vi "verify.vi"(8 "error in":errorcluster, 11 "connection ID":i32) -> (0 "error out":errorcluster, 3 "connection ID":i32)   [LabVIEW 2016]
doc: "Verify that temporary IP configuration is correct"
panel:
  out "params_cluster":cluster{"Numeric":i32}
  in  "Params_cluster":cluster{"Numeric":dbl}
  in  "results_cluster":cluster{"errNo":i32}
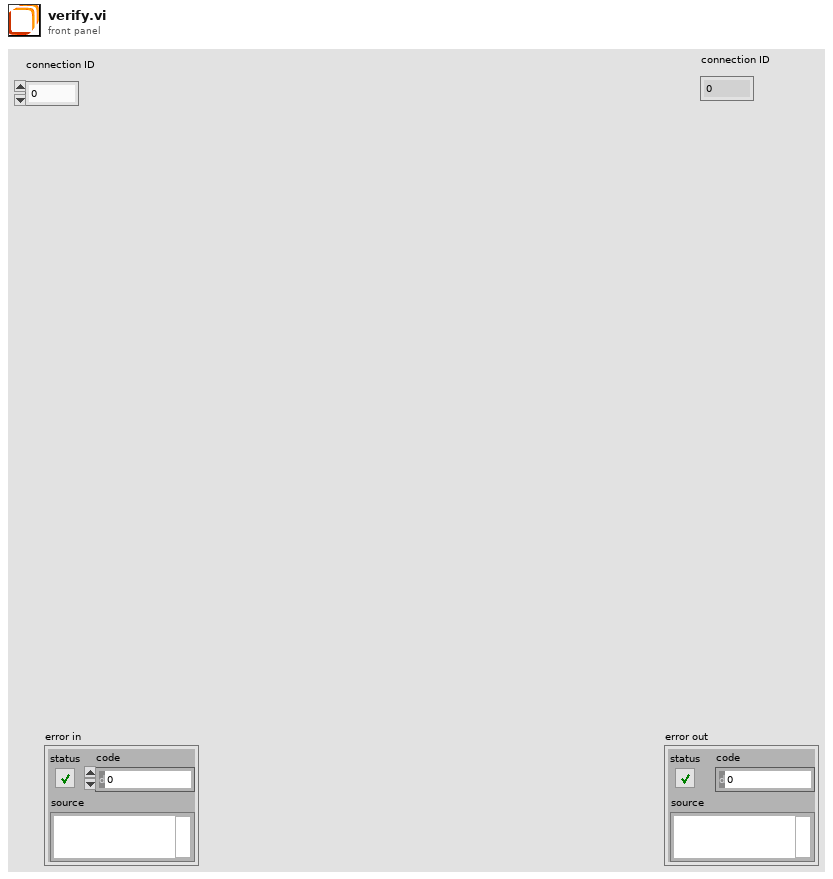
[diagram p1: front panel]
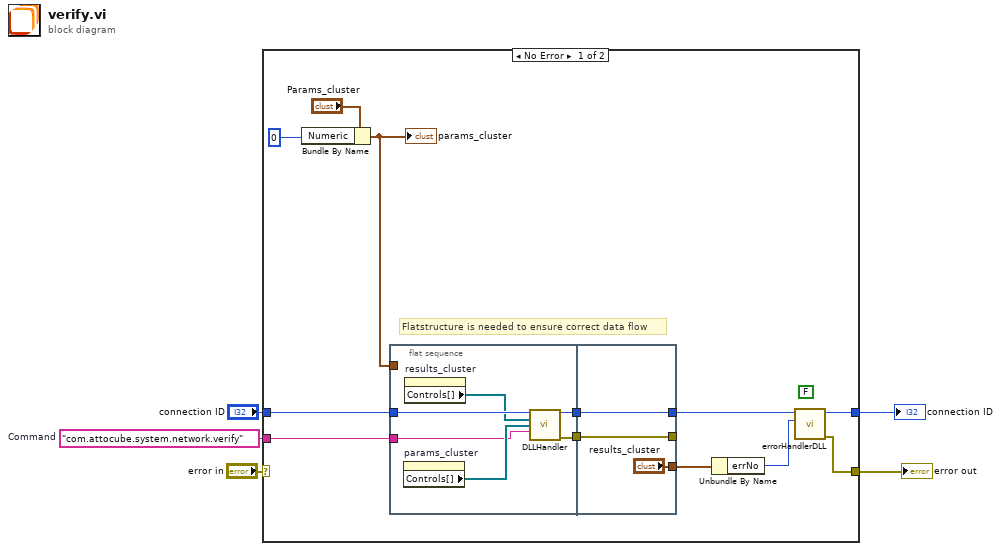
[diagram p0: block diagram]
diagram:
  w3 = "com.attocube.system.network.verify"  # Command
  n1 = case shown="No Error" "error in" {
    selector: "error in" -> [_ w28]
    tunnel: [w7 w28] -> w5
    tunnel: "connection ID" -> [w17 w27]
    tunnel: w3 -> [w14 _]
    tunnel: [w9 w27] -> w1
    frame No Error {
      (unwired) FALSE ("show popup")
      # "Flatstructure is needed to ensure correct data flow"
      n2 = Bundle By Name(cluster="Params_cluster", "Numeric"=0) -> (w12:cluster{"Numeric":dbl})
      "params_cluster" <- w12
      n3 = flat-sequence {
        tunnel: w17 -> [w23]
        tunnel: w14 -> [w20]
        tunnel: [w19] -> w13
        tunnel: w12 -> [_]
        tunnel: [w18] -> w10
        tunnel: ["results_cluster"] -> w16
        tunnel: [w26] -> w11
        tunnel: [w24] -> _
        tunnel: w13 -> [w24]
        tunnel: w10 -> [w26]
        frame #0 {
          n4 = property on="params_cluster" class="Clust (strict)"() -> ("Controls[]"=w21:refnum<vi>[])  [unwired: 2 in, 2 out]
          n5 = property on="results_cluster" class="Clust (strict)"() -> ("Controls[]"=w22:refnum<vi>[])  [unwired: 2 in, 2 out]
          n6 = call "DLLHandler.vi"("connection ID"=w23, "results_cluster"=w22, "params_cluster"=w21, "method"=w20) -> ("connection ID out"=w18:i32, "error"=w19:errorcluster)  [unwired: 10 in]
        }
        frame #1 {
        }
      }
      n7 = Unbundle By Name(w16) -> ("errNo"=w8:i32)
      n8 = call "errorHandlerDLL.vi"("error number"=w8, "connection ID"=w11) -> ("error out"=w7:errorcluster, "connection ID"=w9:i32)  [unwired: 8 in]
    }
    frame Error {
    }
  }
  "error out" <- w5
  "connection ID" <- w1
